vi "Convert_dBm_mW.vi"(1 "Power (dBm)":dbl) -> (0 "Power (mW)":dbl)   [LabVIEW 2020]
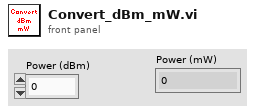
[diagram p1: front panel]
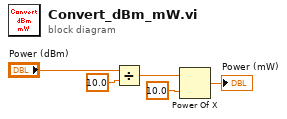
[diagram p0: block diagram]
diagram:
  n1 = Divide(x="Power (dBm)", y=10.0) -> (x/y=w2:dbl)
  n2 = Power Of X(1:10.0 ("y"), 2:w2) -> (0:→"Power (mW)":dbl)
